vi "Send Set Entry Position.vi"(7 "Message Priority (Normal)":T2=enum."Normal", 8 "error in (no error)":errorcluster, 10 "Station":T1, 11 "Message Enqueuer":refnum<class "Message Enqueuer.lvclass">) -> (0 "error out":errorcluster, 3 "Message Enqueuer out":refnum<class "Message Enqueuer.lvclass">)   [LabVIEW 2019, in "Car Wash Controller.lvlib" / "Set Entry Position Msg.lvclass"]
doc: "This VI sends the message to an actor."
uses:
  Set Entry Position Msg.lvclass
  <vilib>/ActorFramework/Message Enqueuer/Message Enqueuer.lvclass
  <vilib>/ActorFramework/Message Enqueuer/Message Priority.ctl
  Vehicle Position Simulation Actor/Car Wash Controller/Station -Enum.ctl
  C:/Program Files (x86)/National Instruments/LabVIEW 2019/vi.lib/ActorFramework/Message/Message.lvclass
  Set Entry Position Msg.lvclass/Set Entry Position Msg.ctl
  <vilib>/ActorFramework/Message Enqueuer/Message Enqueuer.lvclass/Message Enqueuer.ctl
  <vilib>/ActorFramework/Message Priority Queue/Priority Enqueue.vi
  Vehicle Position Simulation Actor/Car Wash Controller/Vehicle Position Simulation Actor.lvclass
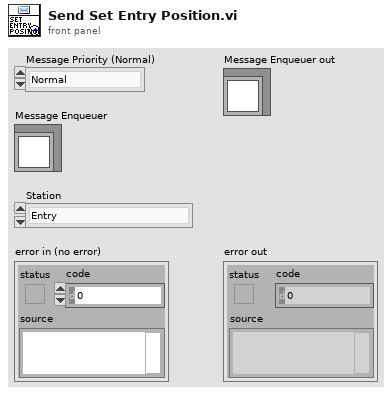
[diagram p1: front panel]
types:
  T1 = typedef "Vehicle Position Sinmulation Actor.lvlib/Vehicle Position Simulation Actor.lvclass/Station -Enum.ctl" = enum16{"Entry", "Station1", "Station2", "Station3", "Exit"}
  T2 = typedef "Actor Framework.lvlib/Message Enqueuer.lvclass/Message Priority.ctl" = enum16{"Low", "Normal", "High"}
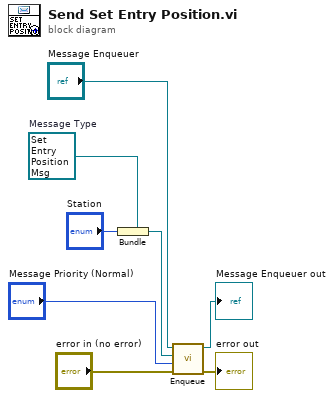
[diagram p0: block diagram]
diagram:
  w5 = refnum<class "Set Entry Position Msg.lvclass"> refnum  # Message Type
  n1 = Bundle(cluster=w5, "Station") -> (w4:refnum<class "Set Entry Position Msg.lvclass">)
  n2 = call <vilib>:"Enqueue.vi"("error in (no error)"="error in (no error)", "Message Priority (Normal)"="Message Priority (Normal)", "Message"=w4, "Message Enqueuer in"="Message Enqueuer") -> ("error out"=→"error out":errorcluster, "Message Enqueuer out"=→"Message Enqueuer out":refnum<class "Message Enqueuer.lvclass">)  [unwired: 6 in]
